vi "Test Point Correspondence.vi"(11 "Test Case In":refnum<class "Correspondence.lvclass">) -> (0 "error out":errorcluster, 3 "Test Case Out":refnum<class "Correspondence.lvclass">)   [LabVIEW 2020, in "test.lvlib" / "Correspondence.lvclass"]
uses:
  Correspondence.lvclass
  C:/Program Files (x86)/National Instruments/LabVIEW 2020/vi.lib/Astemes/LUnit/Test Case.lvclass
  g_pc_toolkit/Correspondence Index.ctl
  g_pc_toolkit/Point Correspondence Params/Point Correspondence Params.lvclass/Point Correspondence Params.ctl
  <vilib>/Astemes/LUnit/Test Case.lvclass/Test Case.ctl
  <vilib>/Analysis/baseanly.llb/A x Vector.vi
  4993e8ee-a06a-463a-9684-69129f64d5ce.vi
  g_pc_toolkit/Point Correspondence Params/Get Params.vi
  <vilib>/Astemes/LUnit/Core/LUnit Test Case/Private/Append Pass Result.vi
  <vilib>/Astemes/LUnit/Core/LUnit Test Case/Private/Append Fail Result.vi
  4993e8ee-a06a-463a-9684-69129f64d5ce.vi/9c5d11cd-9439-4240-a1ee-d9baace9c924.vi
  <vilib>/Astemes/LUnit/Core/LUnit Test Case/Private/Run In UI.vi
  <vilib>/Utility/error.llb/Clear Errors.vi
  <vilib>/Utility/error.llb/Error Cluster From Error Code.vi
  g_pc_toolkit/Point Correspondence Params/Point Correspondence Params.lvclass
  g_pc_toolkit/g_pc_toolkit.lvlib
  <vilib>/Analysis/NI_AALBase.lvlib
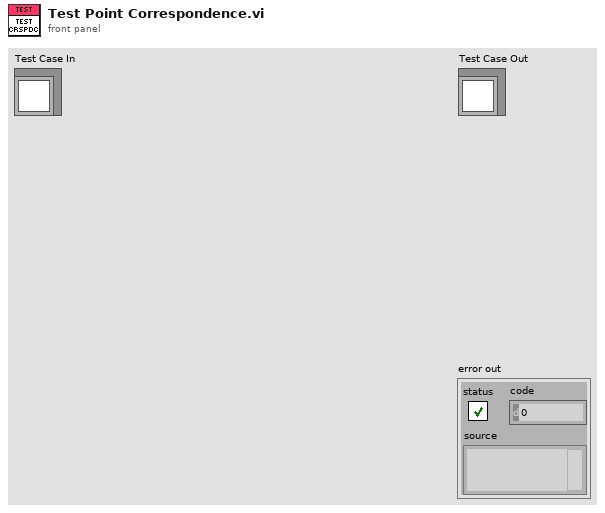
[diagram p1: front panel]
types:
  T1 = typedef "g_pc_toolkit.lvlib/Correspondence Index.ctl" = cluster{"Source Index":i32, "Target Index":i32}
  T2 = cluster{"A x Vector[0]":dbl, "A x Vector[1]":dbl, "A x Vector[2]":dbl}
  T3 = cluster{"A x Vector[0]":dbl, "A x Vector[1]":dbl, "A x Vector[2]":dbl}[]
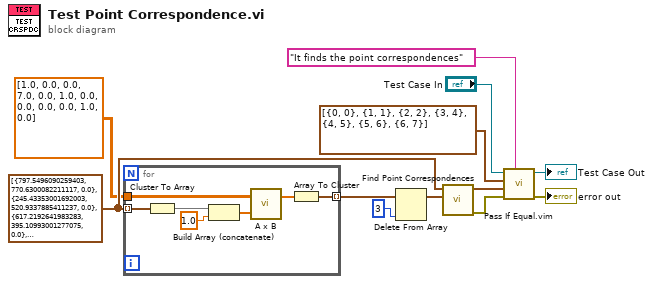
[diagram p0: block diagram]
diagram:
  w9 = cluster{"[0]":dbl, "[1]":dbl, "[2]":dbl}[] [{"[0]"=797.5496090259403, "[1]"=770.6300082211117, "[2]"=0.0}, {"[0]"=245.43353001692003, "[1]"=520.9337885411237, "[2]"=0.0}, {"[0]"=617.2192641983283, "[1]"=395.10993001277075, "[2]"=0.0}, {"[0]"=603.1572496880301, "[1]"=740.1507199512957, "[2]"=0.0}, {"[0]"=879.5232560767754, "[1]"=180.70493783960865, "[2]"=0.0}, {"[0]"=384.34882193321664, "[1]"=801.7026058480797, "[2]"=0.0}, {"[0]"=399.4747322872463, "[1]"=722.1664177342245, "[2]"=0.0}, {"[0]"=206.2512269974468, "[1]"=28.808491846380093, "[2]"=0.0}] ("Array")
  n1 = for {
    tunnel: w9 -> [w19] mode=indexing
    tunnel: [w13] -> w8 mode=indexing
    tunnel: dbl[][] [[1.0, 0.0, 0.0, 7.0], [0.0, 1.0, 0.0, 0.0], [0.0, 0.0, 1.0, 0.0]] -> [w16]
    n2 = Cluster To Array(cluster=w19) -> (array=w18:dbl[])
    n3 = Build Array (concatenate)(w18, 1.0) -> (w15:dbl[])
    n4 = call-poly <vilib>:"A x B.vi"("Vector"=w15, "A"=w16) -> ("A x Vector"=w14:dbl[])  [unwired: 1 out]
    n5 = Array To Cluster(array=w14) -> (cluster=w13:T2)
  }
  n6 = Delete From Array(array=w8, index=3) -> (array with subset deleted=w7:T3)  [unwired: 1 in, 1 out]
  n7 = call "Find Point Correspondences.vi"("Target Points"=w7, "Source Points"=w9) -> ("error out"=w4:errorcluster, "Correspondences"=w1:T1[])  [unwired: 8 in]
  n8 = call "Pass If Equal.vim"("Description"="It finds the point correspondences", "error in (no error)"=w4, "Actual"=w1, "Expected"=T1[] [{"Source Index"=0, "Target Index"=0}, {"Source Index"=1, "Target Index"=1}, {"Source Index"=2, "Target Index"=2}, {"Source Index"=3, "Target Index"=4}, {"Source Index"=4, "Target Index"=5}, {"Source Index"=5, "Target Index"=6}, {"Source Index"=6, "Target Index"=7}] ("Correspondences"), "LUnit Test Case In"="Test Case In") -> ("error out"=→"error out":errorcluster, "LUnit Test Case Out"=→"Test Case Out":refnum<class "Correspondence.lvclass">)  [unwired: 5 in]
